vi "subCreateEventsForStatus.vi"() -> (3 "Events":T1)   [LabVIEW 2020, in "SolutionBuilder.lvlib"]
uses:
  SolutionBuilder.lvlib
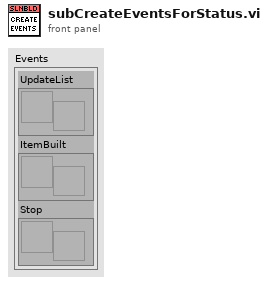
[diagram p1: front panel]
types:
  T1 = cluster{"UpdateList":refnum<user-event>, "ItemBuilt":refnum<user-event>, "Stop":refnum<user-event>}
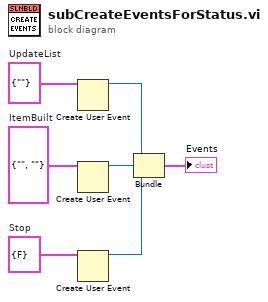
[diagram p0: block diagram]
diagram:
  w5 = cluster{"Item":string} {"Item"=""}  # UpdateList
  w4 = cluster{"Stop":bool} {"Stop"=FALSE}  # Stop
  w3 = cluster{"Item":string, "Result":string} {"Item"="", "Result"=""}  # ItemBuilt
  n1 = Create User Event(user event datatype=w5) -> (user event=w6:refnum<user-event>)  [unwired: 1 in, 1 out]
  n2 = Create User Event(user event datatype=w3) -> (user event=w7:refnum<user-event>)  [unwired: 1 in, 1 out]
  n3 = Create User Event(user event datatype=w4) -> (user event=w2:refnum<user-event>)  [unwired: 1 in, 1 out]
  n4 = Bundle("UpdateList"=w6, "ItemBuilt"=w7, "Stop"=w2) -> (→"Events":T1)  [unwired: 1 in]
